vi "FRCts20_WebMethods_Application_PUT.vi"(6 "query":string, 7 "httpRequestID":u32) -> ()   [LabVIEW 2014]
doc: "<B>PUT</B> on the Application resource\n\n<B>query =</B> archive (default) - Archives team data\n reinitialize - Reintializes the backend\n\nhttp://<server address>:<port>/FRCts/application\n\n{requires authentication}"
uses:
  Backend/source/VI Source/FRCts20_Backend_API/FRCts20_Backend_API_Command_App.ctl
  Backend/source/VI Source/FRCts20_Backend_API/FRCts20_Backend_API_Application.vi
  FRCts20_WebMethods.lvlib
  Backend/source/VI Source/FRCts20_Backend_API/FRCts20_Backend_API.lvlib
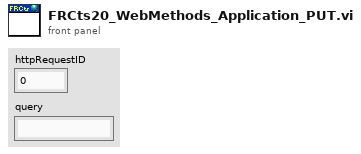
[diagram p1: front panel]
types:
  T1 = typedef "FRCts20_Backend_API.lvlib/FRCts20_Backend_API_Command_App.ctl" = string
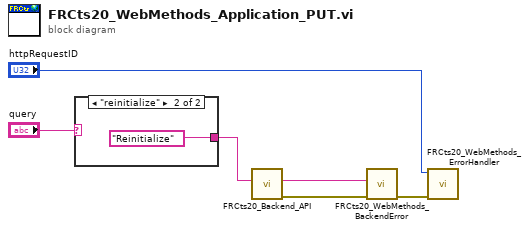
[diagram p0: block diagram]
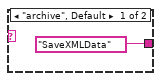
[diagram p2: hidden frame]
diagram:
  n1 = case shown="\"reinitialize\"" "query" {
    tunnel: [T1 "SaveXMLData" ("Command") T1 "Reinitialize" ("Command")] -> w1
    frame "archive", Default {
    }
    frame "reinitialize" {
    }
  }
  n2 = call-poly "FRCts20_Backend_API.vi"("Command"=w1) -> ("error out"=w4:errorcluster, "Status"=w5:string)  [unwired: 8 in, 1 out]
  n3 = call "FRCts20_WebMethods_BackendError.vi"("error in (no error)"=w4, "Status"=w5) -> ("error out"=w3:errorcluster)  [unwired: 8 in, 1 out]
  n4 = call "FRCts20_WebMethods_ErrorHandler.vi"("error in"=w3, "httpRequestID"="httpRequestID") -> ()  [unwired: 9 in, 1 out]
